vi "Parse Object.vi"(8 "error in (no error)":errorcluster, 10 "Index In":i32, 11 "JSON String":string) -> (0 "error out":errorcluster, 2 "Index Out":i32, 3 "JSON Value out":refnum<class "JSON Value.lvclass">)   [LabVIEW 2016, in "JSON Value.lvclass"]
uses:
  JSON Value.lvclass
  subVIs/Errors.ctl
  subVIs/Token Type.ctl
  New JSON Value/New JSON ({Value[]}).vi
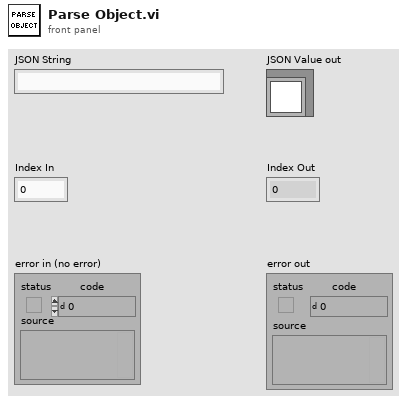
[diagram p1: front panel]
types:
  T1 = typedef "JSON Value.lvclass/Errors.ctl" = enum8{"No key", "Key path type", "Array OOB", "Type Mismatch", "Invalid Token"}
  T2 = typedef "JSON Value.lvclass/Token Type.ctl" = enum8{"NONE", "CURLY_OPEN", "CURLY_CLOSE", "SQUARED_OPEN", "SQUARED_CLOSE", "COLON", "COMMA", "STRING", "NUMBER", "TRUE", "FALSE", "NULL"}
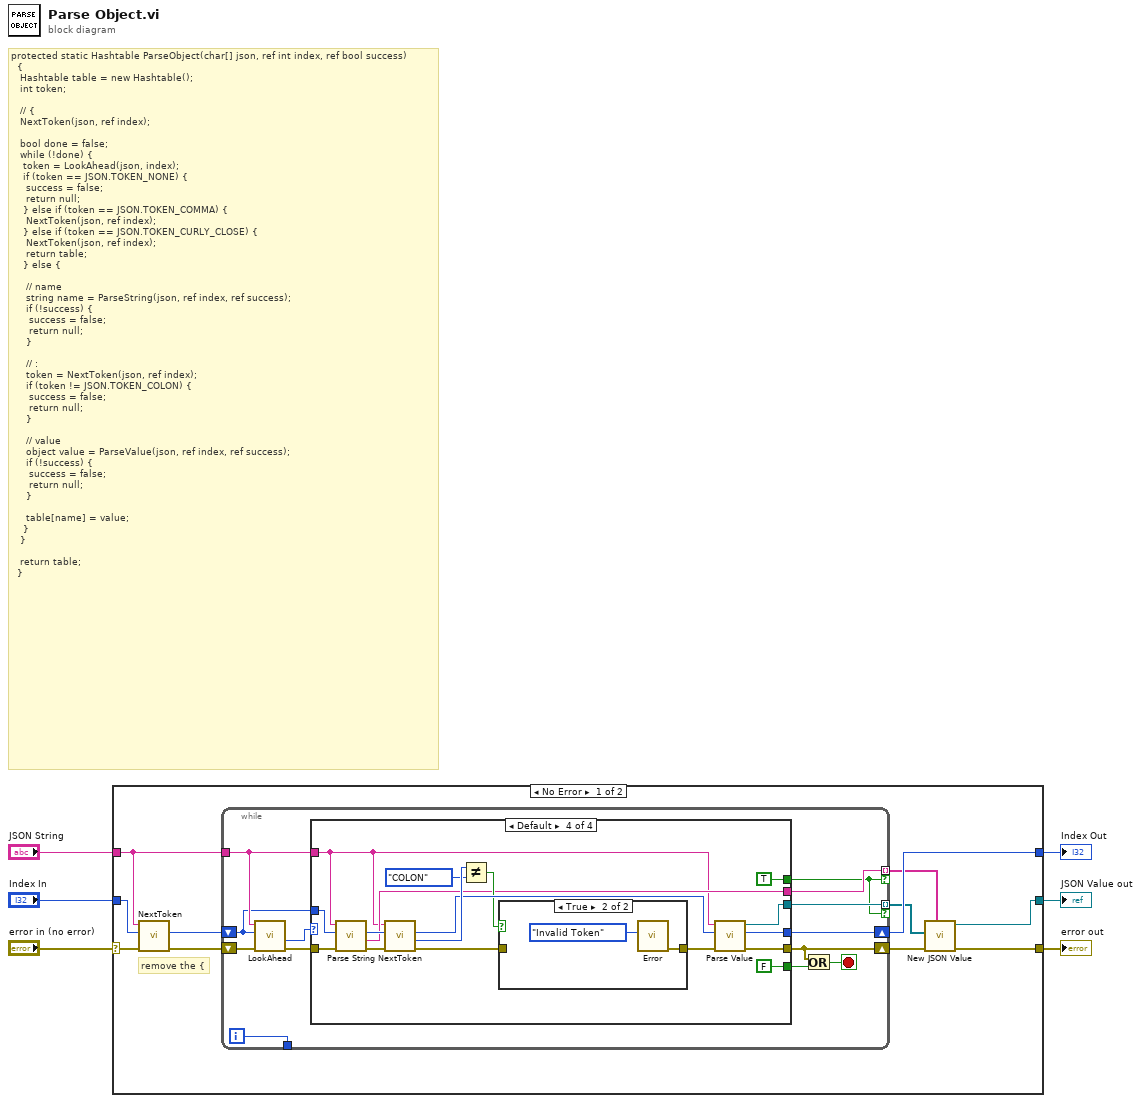
[diagram p0: block diagram]
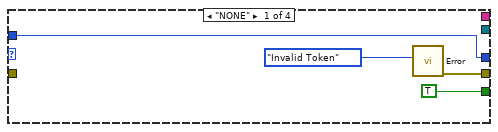
[diagram p2: hidden frame]
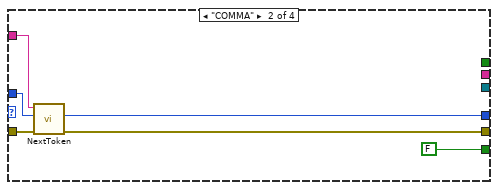
[diagram p3: hidden frame]
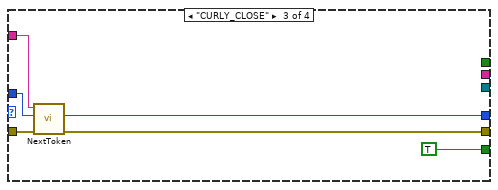
[diagram p4: hidden frame]
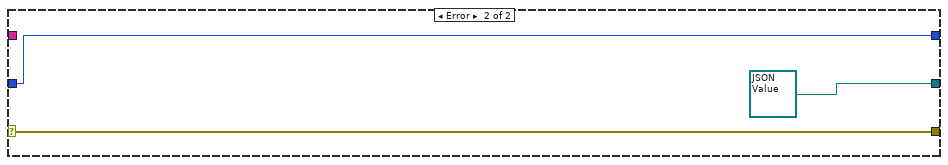
[diagram p6: hidden frame]
diagram:
  # "protected static Hashtable ParseObject(char[] json, ref int index, ref bool success)\n\t\t{\n\t\t\tHashtable table = new Hashtable();\n\t\t\tint token;\n\n\t\t\t// {\n\t\t\tNextToken(json, ref index);\n\n\t\t\tbool done = false;\n\t\t\twhile (!done) {\n\t\t\t\ttoken = LookAhead(json, index);\n\t\t\t\tif (token == JSON.TOKEN_NONE) {\n\t\t\t\t\tsuccess = false;\n\t\t\t\t\treturn null;\n\t\t\t\t} else if (token == JSON.TOKEN_COMMA) {\n\t\t\t\t\tNextToken(json, ref index);\n\t\t\t\t} else if (token == JSON.TOKEN_CURLY_CLOSE) {\n\t\t\t\t\tNextToken(json, ref index);\n\t\t\t\t\treturn table;\n\t\t\t\t} else {\n\n\t\t\t\t\t// name\n\t\t\t\t\tstring name = ParseString(json, ref index, ref success);\n\t\t\t\t\tif (!success) {\n\t\t\t\t\t\tsuccess = false;\n\t\t\t\t\t\treturn null;\n\t\t\t\t\t}\n\n\t\t\t\t\t// :\n\t\t\t\t\ttoken = NextToken(json, ref index);\n\t\t\t\t\tif (token != JSON.TOKEN_COLON) {\n\t\t\t\t\t\tsuccess = false;\n\t\t\t\t\t\treturn null;\n\t\t\t\t\t}\n\n\t\t\t\t\t// value\n\t\t\t\t\tobject value = ParseValue(json, ref index, ref success);\n\t\t\t\t\tif (!success) {\n\t\t\t\t\t\tsuccess = false;\n\t\t\t\t\t\treturn null;\n\t\t\t\t\t}\n\n\t\t\t\t\ttable[name] = value;\n\t\t\t\t}\n\t\t\t}\n\n\t\t\treturn table;\n\t\t}"
  n1 = case shown="No Error" "error in (no error)" {
    selector: "error in (no error)" -> [w13 w68]
    tunnel: [w8 w68] -> w5
    tunnel: "Index In" -> [w14 w69]
    tunnel: [w17 w69] -> w3
    tunnel: [w10 refnum<class "JSON Value.lvclass"> refnum ("JSON Object in")] -> w1
    tunnel: "JSON String" -> [w7 _]
    frame No Error {
      # "remove the {"
      n2 = call "NextToken.vi"("error in (no error)"=w13, "Index In"=w14, "JSON String"=w7) -> ("error out"=w16:errorcluster, "Index Out"=w15:i32)  [unwired: 6 in, 1 out]
      n3 = while {
        tunnel: w7 -> [w20]
        shift-right: [w27] -> w17
        shift-left: w15 -> [w19]
        shift-right: [w24] -> w9
        shift-left: w16 -> [w30]
        tunnel: [w23] -> w12 mode=indexing if=w21
        tunnel: [w22] -> w11 mode=indexing if=w21
        tunnel: [w18] -> _
        i -> [w18]
        stop <- w25 stop-if-true
        n4 = call "LookAhead.vi"("error in (no error)"=w30, "Index"=w19, "JSON String"=w20) -> ("error out"=w28:errorcluster, "TOKEN"=w29:T2)  [unwired: 7 in]
        n5 = case shown="Default" w29 {
          tunnel: [TRUE FALSE TRUE FALSE] -> w26
          tunnel: w28 -> [_ w40 w46 w63]
          tunnel: [w32 w37 w43 w55] -> w24
          tunnel: w19 -> [w33 w39 w45 w62]
          tunnel: [w33 w38 w44 w56] -> w27
          tunnel: w20 -> [_ w35 w41 w47]
          tunnel: [_ _ _ w48] -> w23
          tunnel: [_ _ _ w50] -> w22
          tunnel: [_ _ _ TRUE] -> w21
          frame "NONE" {
            n6 = call "Error.vi"("Error"=Errors."Invalid Token") -> ("error out"=w32:errorcluster)  [unwired: 9 in]
          }
          frame "COMMA" {
            n7 = call "NextToken.vi"("error in (no error)"=w40, "Index In"=w39, "JSON String"=w35) -> ("error out"=w37:errorcluster, "Index Out"=w38:i32)  [unwired: 6 in, 1 out]
          }
          frame "CURLY_CLOSE" {
            n8 = call "NextToken.vi"("error in (no error)"=w46, "Index In"=w45, "JSON String"=w41) -> ("error out"=w43:errorcluster, "Index Out"=w44:i32)  [unwired: 6 in, 1 out]
          }
          frame Default {
            n9 = call "Parse String.vi"("error in (no error)"=w63, "Index In"=w62, "JSON String"=w47) -> ("error out"=w61:errorcluster, "Parsed String"=w48:string, "Index Out"=w60:i32)  [unwired: 5 in, 1 out]
            n10 = call "NextToken.vi"("error in (no error)"=w61, "Index In"=w60, "JSON String"=w47) -> ("error out"=w51:errorcluster, "TOKEN"=w59:T2, "Index Out"=w57:i32)  [unwired: 6 in]
            n11 = Not Equal?(x=w59, y=Token_Type."COLON") -> (x != y?=w53:bool)
            n12 = case shown="True" w53 {
              tunnel: [w64 w65] -> w52
              tunnel: w51 -> [w64 _]
              frame False {
              }
              frame True {
                n13 = call "Error.vi"("Error"=Errors."Invalid Token") -> ("error out"=w65:errorcluster)  [unwired: 9 in]
              }
            }
            n14 = call "Parse Value.vi"("error in (no error)"=w52, "Index In"=w57, "JSON String"=w47) -> ("error out"=w55:errorcluster, "Index Out"=w56:i32, "JSON Value out"=w50:refnum<class "JSON Value.lvclass">)  [unwired: 6 in]
          }
        }
        n15 = Or(x=w24, y=w26) -> (x .or. y?=w25:bool)
      }
      n16 = call-poly "New JSON Value.vi"("keys"=w12, "error in (no error)"=w9, "values"=w11) -> ("error out"=w8:errorcluster, "JSON Value out"=w10:refnum<class "JSON Value.lvclass">)  [unwired: 7 in]
    }
    frame Error {
    }
  }
  "error out" <- w5
  "Index Out" <- w3
  "JSON Value out" <- w1
